vi "Timestamper Start Message.vi"(8 "error in (no error)":errorcluster, 11 "AcquistionObject in":refnum<class "AcquistionObject.lvclass">) -> (0 "error out":errorcluster, 3 "AcquistionObject out":refnum<class "AcquistionObject.lvclass">)   [LabVIEW 2010, in "AcquistionObject.lvclass"]
uses:
  AcquistionObject.lvclass
  AcquistionObject.lvclass/AcquistionObject.ctl
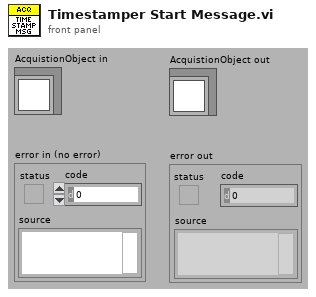
[diagram p1: front panel]
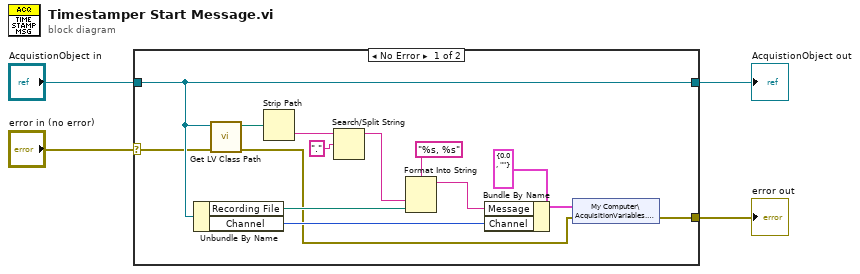
[diagram p0: block diagram]
diagram:
  n1 = case shown="No Error" "error in (no error)" {
    selector: "error in (no error)" -> [w6 w20]
    tunnel: [w5 w20] -> w3
    tunnel: [w12 w19] -> w1
    tunnel: "AcquistionObject in" -> [w12 w19]
    frame No Error {
      n2 = Unbundle By Name(w12) -> ("Recording File"=w11:path, "Channel"=w14:i16)
      n3 = call <vilib>:"Get LV Class Path.vi"("error in (no error)"=w6, "object"=w12) -> ("error out"=w7:errorcluster, "class path"=w13:path)  [unwired: 8 in]
      n4 = Strip Path(path=w13) -> (name=w9:string)  [unwired: 1 out]
      n5 = Search/Split String(string=w9, search string/char (-)=".") -> (substring before match=w8:string)  [unwired: 1 in, 2 out]
      n6 = Format Into String(format string="%s, %s", w8, w11) -> (resulting string=w15:string)  [unwired: 2 in, 1 out]
      n7 = Bundle By Name(cluster=cluster{"Channel":dbl, "Message":string} {"Channel"=0.0, "Message"=""} ("Message"), "Message"=w15, "Channel"=w14) -> (w18:cluster{"Channel":dbl, "Message":string})
      n8 = shared-variable "My Computer\\AcquisitionVariables.lvlib\\Message"(w18, error in=w7) -> (error out=w5:errorcluster)
    }
    frame Error {
    }
  }
  "error out" <- w3
  "AcquistionObject out" <- w1
